vi "AnalogOutput.vi"(8 "Output array":i32[](array[numeric])=[0, 0, 0, 0, 0, 0, 0, 0], 10 "Analog output":dbl, 11 "Output Channel":T1(ring)) -> (0 "Updated output array":i32[](array[numeric]))   [LabVIEW 2025]
doc: "Inserts analog output value into analog output \narray in preperation for write to MB server.\nIf output array input is unwired, output array\nis initialised as 8x1 array of type int.\n\nINPUTS:\n 1. Analog output channel -- int 0-7 or auto\n configured enum AO-0 -> AO-7\n 2. Anlog output value -- DBL\n 3. Array of values to write to MB server.\n int array with dimension 8x1\n\nOUTPUTS:\n 1. Array of values to write to MB server\n int with dimension 8x1. -- updated array\n obtained from input 2"
panel:
  # "Write single analog output to output array\n\nInserts analog output value into analog output \narray in preperation for write to MB server.\nIf output array input is unwired, output array\nis initialised as 8x1 array of type int.\n\nINPUTS:\n  1. Analog output channel -- int 0-7 or auto\n      configured enum AO-0 -> AO-7\n  2. Anlog output value -- DBL\n  3. Array of values to write to MB server.\n       int array with dimension 8x1\n\nOUTPUTS:\n   1. Array of values to write to MB server\n       int with dimension 8x1. -- updated array\n       obtained from input 2"
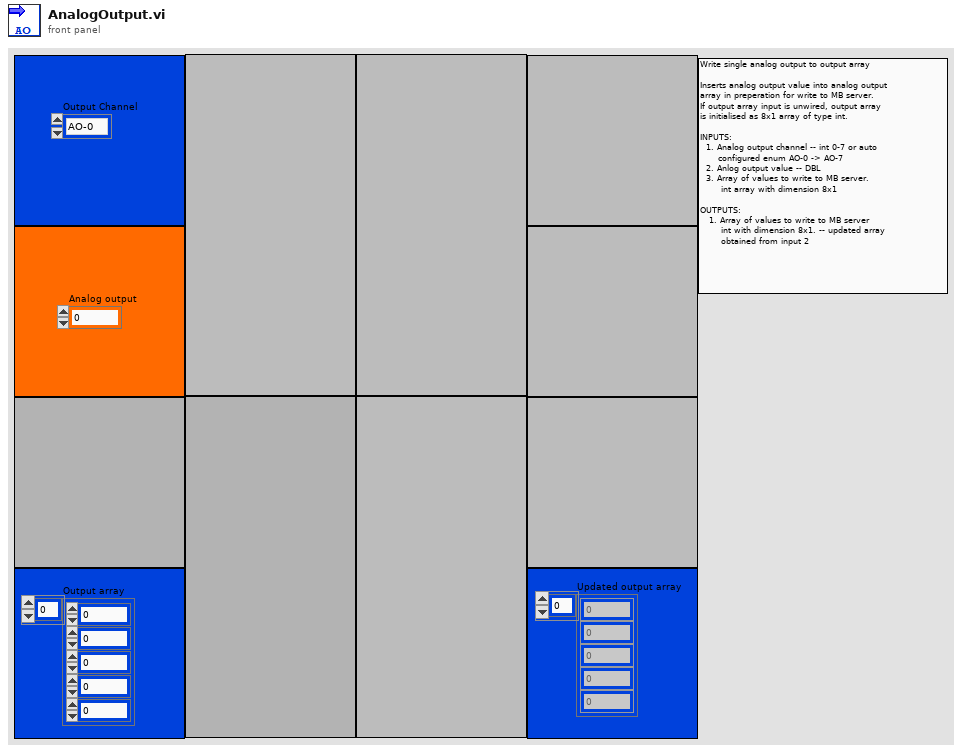
[diagram p1: front panel]
types:
  T1 = enum16{"AO-0", "AO-1", "AO-2", "AO-3", "AO-4", "AO-5", "AO-6", "AO-7"}
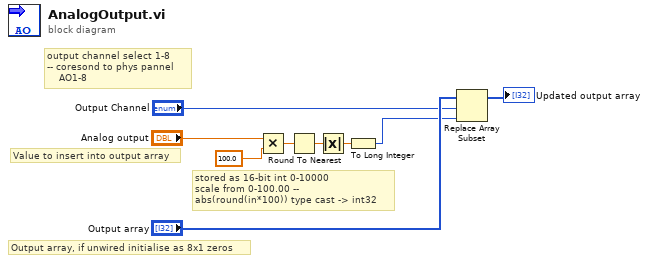
[diagram p0: block diagram]
diagram:
  # "stored as 16-bit int 0-10000\nscale from 0-100.00 --\nabs(round(in*100)) type cast -> int32"
  # "Output array, if unwired initialise as 8x1 zeros"
  # "Value to insert into output array"
  # "output channel select 1-8\n-- coresond to phys pannel\n    AO1-8"
  n1 = Multiply(x="Analog output", y=100.0) -> (x*y=w6:dbl)
  n2 = Round To Nearest(number=w6) -> (nearest integer value=w8:dbl)
  n3 = Absolute Value(x=w8) -> (abs(x)=w9:dbl)
  n4 = To Long Integer(number=w9) -> (32bit integer=w3:i32)
  n5 = Replace Array Subset(array="Output array", new element=w3, index="Output Channel") -> (→"Updated output array":i32[])
